vi "Mcp2210 Get Access Ctrl Status.vi"(8 "error in (no error)":errorcluster, 11 "handle":i32) -> (0 "error out":errorcluster, 1 "Password Attempt Count":u8, 2 "NVRAM Access Control":u8(ring) items=["No protected"=0, "Protected by Password"=40, "Permanently Locked"=80], 3 "handle out":i32, 4 "Password accept":u16(ring) items=["Not Accepted", "Accepted"])   [LabVIEW 2015, in "mcp2210.lvlib"]
doc: "This command provides information about the NVARM access control status.\nIn case of successful execution, the function returns 0 (E_SUCCESS) and updates the pointer\nparameters with the status codes. In case of failure, negative error code is returned.\nParameters:\nInputs:\n- void *handle - The pointer to the USB device handle. Cannot be NULL.\nOutputs:\n- unsigned char *pAccessCtrl - NVRAM chip settings access control:\n- 0x00 - settings not protected\n- 0x40 - settings protected by Password\n- 0x80 - settings permanently locked\nParameter cannot be NULL.\n- unsigned char *pPasswdAttemptCnt - counts how many times the NVRAM password was tried.\nThe value will saturate to 5 even if the number of wrong\nattempts exceeds 5. After the password is accepted, the\ncounter is reset to 0.\nParameter cannot be NULL.\n- unsigned char *pPasswdAccepted - If the NVRAM access is password protected\n(indicated by *pAccessCtrl == 0x40), this flag indicates\nwhether the password has been accepted or not after using the\nMcp2210_EnterAccessPasswd() command:\n- 0x00 - Password NOT accepted\n- 0x01 - Password accepted.\n- If the NVRAM access is not password protected\n(indicated by *pAccessCtrl == 0x00), this flag returns 0x00.\nThe parameter cannot be NULL.\nReturns:\n- 0 for success: E_SUCCESS\n- negative error code: E_ERR_NULL, E_ERR_INVALID_HANDLE_VALUE\nE_ERR_HID_TIMEOUT, E_ERR_HID_RW_FILEIO, E_ERR_UNKOWN_ERROR\nE_ERR_CMD_ECHO, E_ERR_CMD_FAILED\n\nMCP2210_DLL_UM_API int __stdcall Mcp2210_GetAccessCtrlStatus(void *handle, unsigned char *pAccessCtrl, unsigned char *pPasswdAttemptCnt, unsigned char *pPasswdAccepted);"
uses:
  <userlib>/mcp2210/mcp2210.lvlib
  <userlib>/mcp2210/mcp2210_dll_um_x86.dll
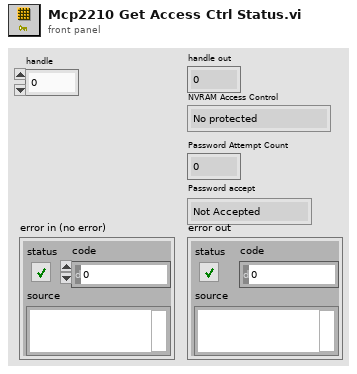
[diagram p1: front panel]
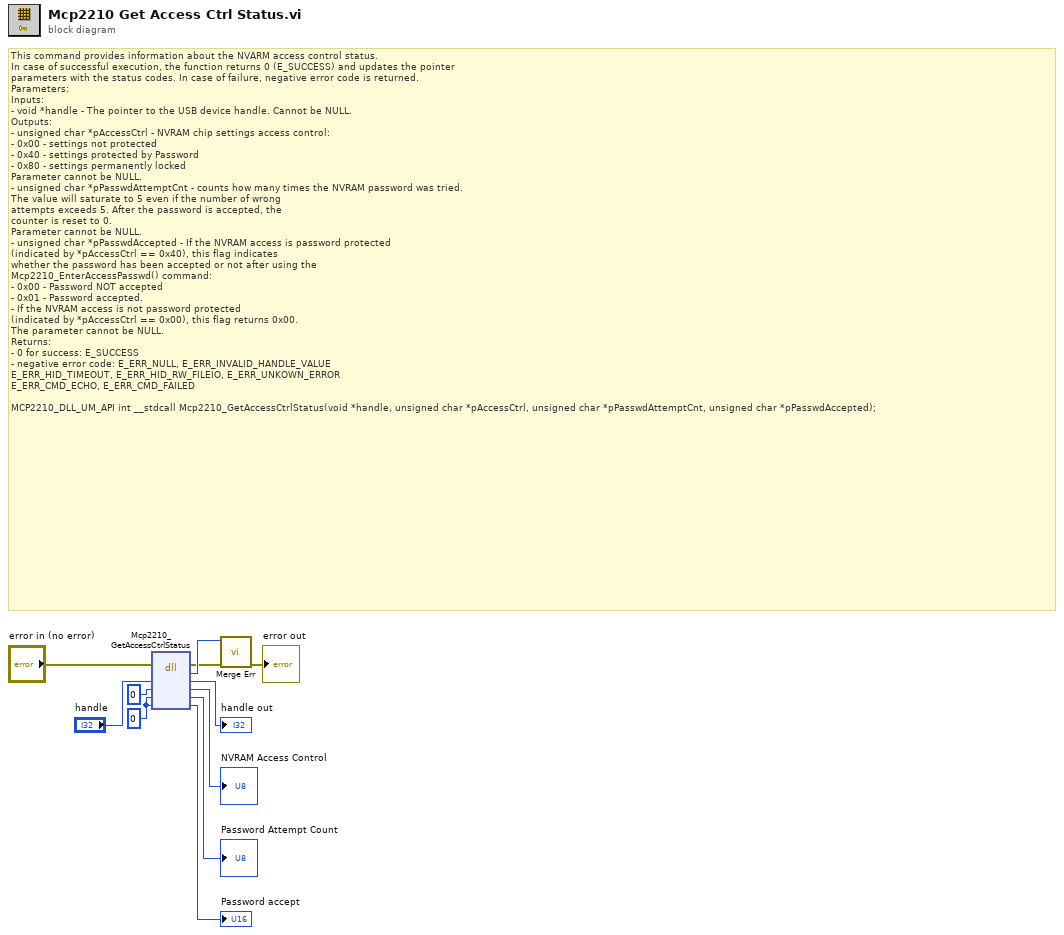
[diagram p0: block diagram]
diagram:
  w2 = u8 0 ("pPasswdAttemptCnt")
  # "This command provides information about the NVARM access control status.\nIn case of successful execution, the function returns 0 (E_SUCCESS) and updates the pointer\nparameters with the status codes. In case of failure, negative error code is returned.\nParameters:\nInputs:\n- void *handle - The pointer to the USB device handle. Cannot be NULL.\nOutputs:\n- unsigned char *pAccessCtrl - NVRAM chip settings access control:\n- 0x00 - settings not protected\n- 0x40 - settings protected by Password\n- 0x80 - settings permanently locked\nParameter cannot be NULL.\n- unsigned char *pPasswdAttemptCnt - counts how many times the NVRAM password was tried.\nThe value will saturate to 5 even if the number of wrong\nattempts exceeds 5. After the password is accepted, the\ncounter is reset to 0.\nParameter cannot be NULL.\n- unsigned char *pPasswdAccepted - If the NVRAM access is password protected\n(indicated by *pAccessCtrl == 0x40), this flag indicates\nwhether the password has been accepted or not after using the\nMcp2210_EnterAccessPasswd() command:\n- 0x00 - Password NOT accepted\n- 0x01 - Password accepted.\n- If the NVRAM access is not password protected\n(indicated by *pAccessCtrl == 0x00), this flag returns 0x00.\nThe parameter cannot be NULL.\nReturns:\n- 0 for success: E_SUCCESS\n- negative error code: E_ERR_NULL, E_ERR_INVALID_HANDLE_VALUE\nE_ERR_HID_TIMEOUT, E_ERR_HID_RW_FILEIO, E_ERR_UNKOWN_ERROR\nE_ERR_CMD_ECHO, E_ERR_CMD_FAILED\n\nMCP2210_DLL_UM_API int __stdcall Mcp2210_GetAccessCtrlStatus(void *handle, unsigned char *pAccessCtrl, unsigned char *pPasswdAttemptCnt, unsigned char *pPasswdAccepted);"
  n1 = dll-call lib="D:/LabVIEW 2015/user.lib/mcp2210/mcp2210_dll_um_x86.*" fn="Mcp2210_GetAccessCtrlStatus"(error in="error in (no error)", "handle"="handle", "pAccessCtrl"=u8 0, "pPasswdAttemptCnt"=w2, "pPasswdAccepted"=w2) -> (error out=w7:errorcluster, "return type"=w8:i32, "handle"=→"handle out":i32, "pAccessCtrl"=→"NVRAM Access Control":u8, "pPasswdAttemptCnt"=→"Password Attempt Count":u8, "pPasswdAccepted"=→"Password accept":u8)  [unwired: 2 in, 1 out]
  n2 = call <userlib>:"Merge Err.vi"("error in (no error)"=w7, "return type"=w8) -> ("error out"=→"error out":errorcluster)  [unwired: 9 in]
